vi "FTW-Supervisor-Core-LogSchema.vi"() -> (6 "Schema":string, 10 "Indexes":string)   [LabVIEW 2014, in "FTW-Supervisor.lvclass"]
uses:
  FTW-Supervisor.lvclass
panel:
  # "Outputs"
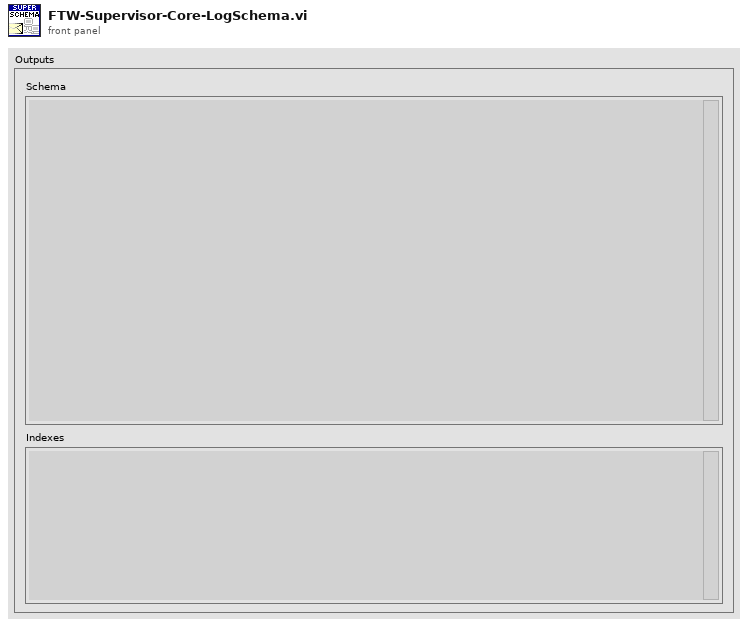
[diagram p1: front panel]
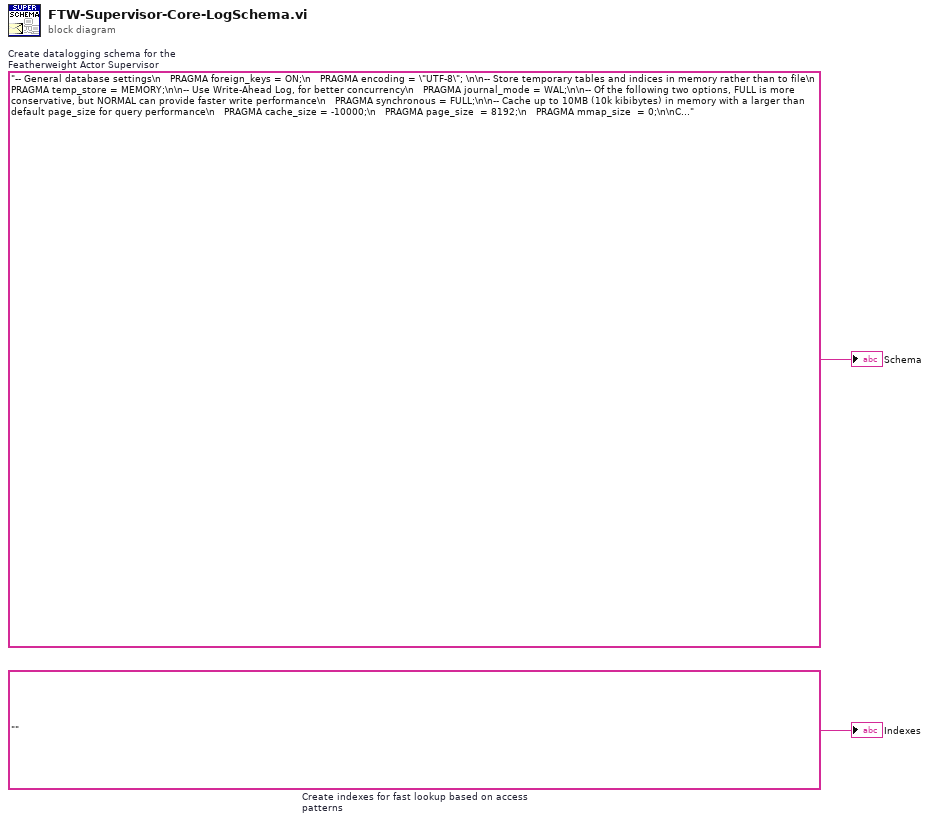
[diagram p0: block diagram]
diagram:
  w1 = ""  # Create indexes for fast lookup based on access patterns
  w2 = "-- General database settings\n   PRAGMA foreign_keys = ON;\n   PRAGMA encoding = \"UTF-8\"; \n\n-- Store temporary tables and indices in memory rather than to file\n   PRAGMA temp_store = MEMORY;\n\n-- Use Write-Ahead Log, for better concurrency\n   PRAGMA journal_mode = WAL;\n\n-- Of the following two options, FULL is more conservative, but NORMAL can provide faster write performance\n   PRAGMA synchronous = FULL;\n\n-- Cache up to 10MB (10k kibibytes) in memory with a larger than default page_size for query performance\n   PRAGMA cache_size = -10000;\n   PRAGMA page_size  = 8192;\n   PRAGMA mmap_size  = 0;\n\nCREATE TABLE IF NOT EXISTS settings (\n  key   TEXT PRIMARY KEY,\n  value\n);\n\nCREATE TABLE IF NOT EXISTS application (\n  id                INTEGER PRIMARY KEY AUTOINCREMENT,\n  name              TEXT,\n  version_major     INTEGER,\n  version_minor     INTEGER,\n  version_patch     INTEGER,\n  UNIQUE            (name, version_major, version_minor, version_patch) ON CONFLICT IGNORE\n);\n\nCREATE TABLE IF NOT EXISTS session (\n  id                  INTEGER PRIMARY KEY AUTOINCREMENT,\n  application_id      INTEGER REFERENCES application(id) NOT NULL,\n  timestamp_started   REAL NOT NULL,\n  timestamp_stopped   REAL NOT NULL\n);\n\nCREATE TABLE IF NOT EXISTS actor (\n  id                  INTEGER PRIMARY KEY AUTOINCREMENT,\n  application_id      INTEGER REFERENCES application(id) NOT NULL,\n  name                TEXT,\n  UNIQUE              (application_id, name) ON CONFLICT IGNORE\n);\n\nCREATE TABLE IF NOT EXISTS eventDefinition (\n  id                  INTEGER PRIMARY KEY AUTOINCREMENT,\n  type                TEXT,\n  code                TEXT,\n  UNIQUE              (type, code) ON CONFLICT IGNORE\n);\n\nCREATE TABLE IF NOT EXISTS channelDefinition (\n  id       INTEGER PRIMARY KEY AUTOINCREMENT,\n  name     TEXT,\n  UNIQUE   (name) ON CONFLICT IGNORE\n);\n\nCREATE TABLE IF NOT EXISTS channelData (\n  timestamp     REAL NOT NULL,\n  channel_id    INTEGER REFERENCES channelDefinition(id) NOT NULL DEFERRABLE INITIALLY DEFERRED,\n  value,\n  PRIMARY KEY (timestamp, channel_id)\n);\n\nCREATE TABLE IF NOT EXISTS eventData (\n  id       INTEGER PRIMARY KEY AUTOINCREMENT,\n  data     UNIQUE\n);\n\nCREATE TABLE IF NOT EXISTS event (\n  session_id    INTEGER REFERENCES session(id) NOT NULL DEFERRABLE INITIALLY DEFERRED,\n  actor_id      INTEGER REFERENCES actor(id) NOT NULL DEFERRABLE INITIALLY DEFERRED,\n  data_id       INTEGER REFERENCES eventData(id) NOT NULL DEFERRABLE INITIALLY DEFERRED,\n  timestamp     REAL NOT NULL\n);"  # Create datalogging schema for the Featherweight Actor Supervisor
  "Schema" <- w2
  "Indexes" <- w1
